vi "save_T1_no-dialog.vi"(5 "triggers":u32[][](array[numeric]), 6 "file_path":path, 7 "timetags":u32[][](array[numeric]), 8 "fitted_signal_in":T2 caption="fitted_signal", 9 "fit_parameters":T4 {"T1 2" format="%.3g"; "T1" format="%.3g"; "C1" format="%.3g"; "Tm" format="%.3g"; "Cm" format="%.3g"; "Ie" format="%.3g"}, 10 "T1_parameters":T1, 11 "T1_curve_in":T3) -> (0 "error out":errorcluster)   [LabVIEW 2014]
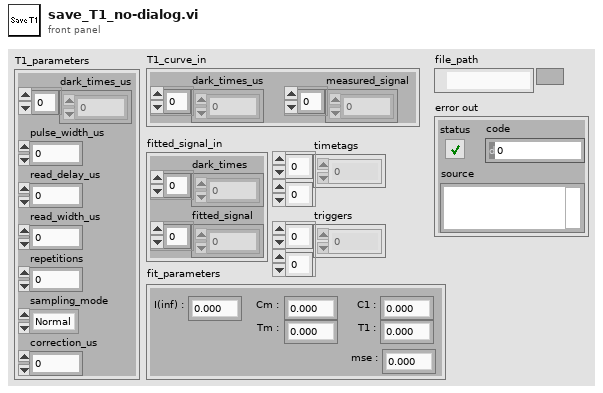
[diagram p1: front panel]
types:
  T1 = cluster{"dark_times_us":dbl[], "pulse_width_us":dbl, "read_delay_us":dbl, "read_width_us":dbl, "repetitions":i32, "sampling_mode":enum16{"Normal", "Sweep"}, "correction_us":dbl}
  T2 = cluster{"dark_times":dbl[], "fitted_signal":dbl[]}
  T3 = cluster{"dark_times_us":dbl[], "measured_signal":dbl[]}
  T4 = cluster{"Ie":dbl, "Cm":dbl, "Tm":dbl, "C1":dbl, "T1":dbl, "T1 2":dbl}
  T5 = enum16{"open", "replace", "create", "open or create", "replace or create", "replace or create with confirmation"}
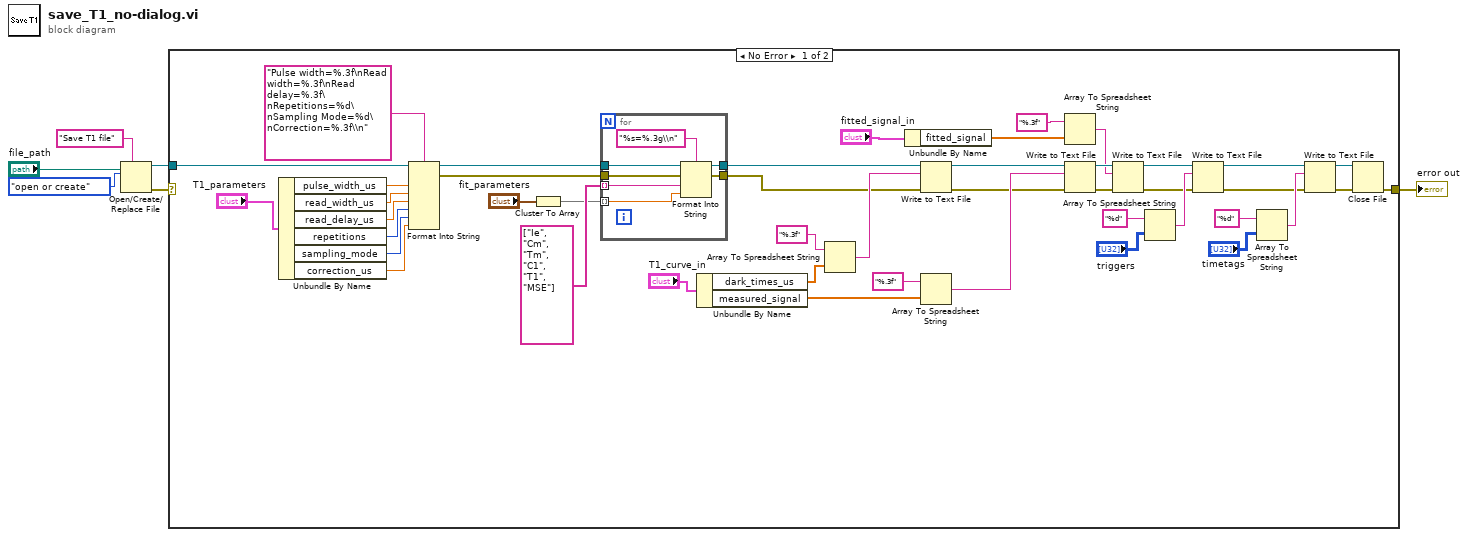
[diagram p0: block diagram]
diagram:
  n1 = Open/Create/Replace File(file path (use dialog)="file_path", prompt="Save T1 file", operation (0:open)=T5."open or create") -> (refnum out=w5:refnum<file>, error out=w3:errorcluster)  [unwired: 3 in, 1 out]
  n2 = case shown="No Error" w3 {
    selector: w3 -> [_ w58]
    tunnel: w5 -> [w15 _]
    tunnel: [w7 w58] -> w1
    frame No Error {
      n3 = Unbundle By Name("T1_parameters") -> ("pulse_width_us"=w36:dbl, "read_width_us"=w35:dbl, "read_delay_us"=w34:dbl, "repetitions"=w33:i32, "sampling_mode"=w23:enum16{"Normal", "Sweep"}, "correction_us"=w22:dbl)
      n4 = Format Into String(format string="Pulse width=%.3f\nRead width=%.3f\nRead delay=%.3f\nRepetitions=%d\nSampling Mode=%d\nCorrection=%.3f\\n", initial string=w15, w36, w35, w34, w33, w23, w22) -> (resulting string=w16:refnum<file>, error out=w8:errorcluster)  [unwired: 1 in]
      n5 = Cluster To Array(cluster="fit_parameters") -> (array=w48:dbl[])
      n6 = for {
        tunnel: string[] ["Ie", "Cm", "Tm", "C1", "T1", "MSE"] -> [w56] mode=indexing
        tunnel: w48 -> [w55] mode=indexing
        tunnel: [w54] -> w32
        tunnel: w16 -> [w53]
        tunnel: [w52] -> w9
        tunnel: w8 -> [w51]
        n7 = Format Into String(format string="%s=%.3g\\n", initial string=w53, error in=w51, w56, w55) -> (resulting string=w54:refnum<file>, error out=w52:errorcluster)
      }
      n8 = Unbundle By Name("T1_curve_in") -> ("dark_times_us"=w46:dbl[], "measured_signal"=w42:dbl[])
      n9 = Array To Spreadsheet String(array=w46, 3:"%.3f" ("format string")) -> (spreadsheet string=w29:string)  [unwired: 1 in]
      n10 = Unbundle By Name("fitted_signal_in") -> ("fitted_signal"=w41:dbl[])
      n11 = Write to Text File(file (use dialog)=w32, text=w29, error in=w9) -> (refnum out=w44:refnum<file>, error out=w10:errorcluster)  [unwired: 1 in, 1 out]
      n12 = Array To Spreadsheet String(array=w42, 3:"%.3f" ("format string")) -> (spreadsheet string=w31:string)  [unwired: 1 in]
      n13 = Array To Spreadsheet String(array=w41, 3:"%.3f" ("format string")) -> (spreadsheet string=w30:string)  [unwired: 1 in]
      n14 = Write to Text File(file (use dialog)=w44, text=w31, error in=w10) -> (refnum out=w39:refnum<file>, error out=w14:errorcluster)  [unwired: 1 in, 1 out]
      n15 = Write to Text File(file (use dialog)=w39, text=w30, error in=w14) -> (refnum out=w20:refnum<file>, error out=w13:errorcluster)  [unwired: 1 in, 1 out]
      n16 = Array To Spreadsheet String(array="triggers", 3:"%d" ("format string")) -> (spreadsheet string=w18:string)  [unwired: 1 in]
      n17 = Write to Text File(file (use dialog)=w20, text=w18, error in=w13) -> (refnum out=w19:refnum<file>, error out=w12:errorcluster)  [unwired: 1 in, 1 out]
      n18 = Array To Spreadsheet String(array="timetags", 3:"%d" ("format string")) -> (spreadsheet string=w27:string)  [unwired: 1 in]
      n19 = Write to Text File(file (use dialog)=w19, text=w27, error in=w12) -> (refnum out=w28:refnum<file>, error out=w11:errorcluster)  [unwired: 1 in, 1 out]
      n20 = Close File(refnum=w28, error in=w11) -> (error out=w7:errorcluster)  [unwired: 1 out]
    }
    frame Error {
    }
  }
  "error out" <- w1
